vi "TWM Measure.vi"(4 "TWM Status ref":refnum<vi>, 6 "TWM pipe":string, 8 "error in (no error)":errorcluster, 10 "TWM Measurement properties":T1={"Sampling frequency (Hz)"=500000.0, "Record length (multiples of period)"=1000.0, "Signal amplitude (V)"=4.5, "Measurement frequency (Hz)"=1000.0, "Calculate RMS from samples"=FALSE, "Algorithm"="TWM-WFFT", "Quantity"="rms", "Measurement path"=""} {"Measurement frequency (Hz)" format="%#_3p"; "Record length (multiples of period)" format="%#_3p"; "Sampling frequency (Hz)" format="%#_3p"}, 11 "TWM handle":i32) -> (0 "error out":errorcluster, 1 "TWM result as number":dbl[][](array[numeric]), 2 "TWM result as string":string[][](array[string]), 3 "TWM handle out":i32)   [LabVIEW 2020]
doc: "Set TWM measurement, initiate TWM measurement, wait for results if needed, reset connection if error."
uses:
  Type definitions/Sampling properties.ctl
  external libraries/TWM-1.8.7.0-client/TWM Client Quantity Record.ctl
  external libraries/TWM-1.8.7.0-client/TWM Client.lvlib
  external libraries/varilib/varilib.lvlib
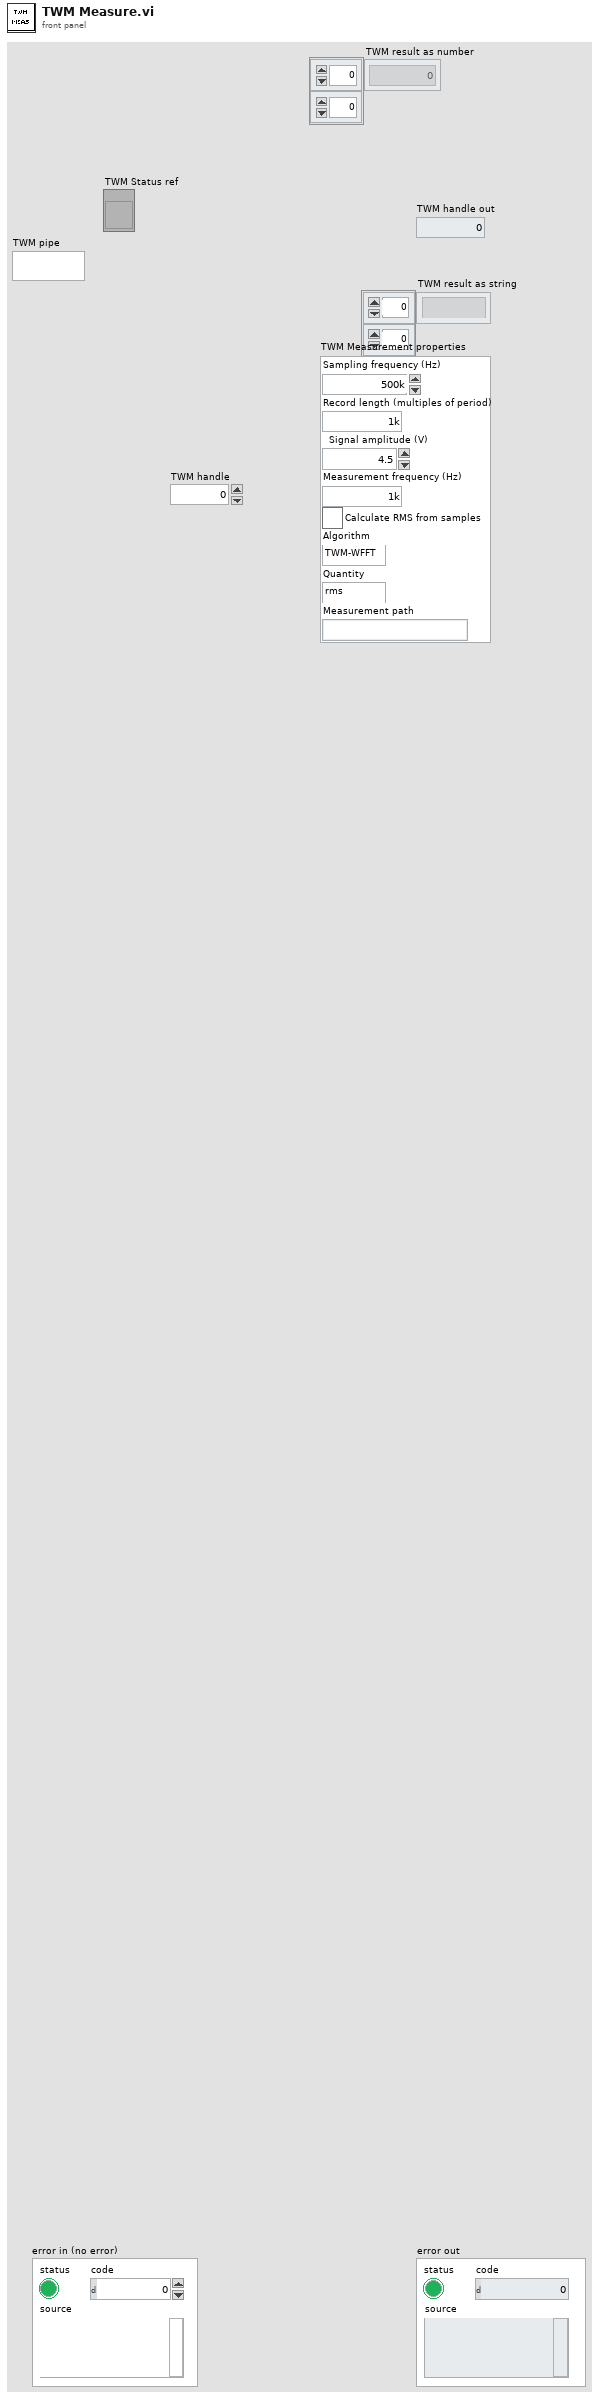
[diagram p1: front panel]
types:
  T1 = typedef "Sampling properties.ctl" = cluster{"Sampling frequency (Hz)":dbl, "Record length (multiples of period)":dbl, "Signal amplitude (V)":dbl, "Measurement frequency (Hz)":dbl, "Calculate RMS from samples":bool, "Algorithm":string, "Quantity":string, "Measurement path":string}
  T2 = typedef "TWM Client.lvlib/TWM Client Quantity Record.ctl" = cluster{"val":dbl[], "unc":dbl[], "name":string, "is valid?":bool, "has unc?":bool, "numel":i32, "ua":dbl[], "is phase?":bool, "is amplitude?":bool, "description":string, "phase tag":string, "num format":string, "is string?":bool, "string value":string}
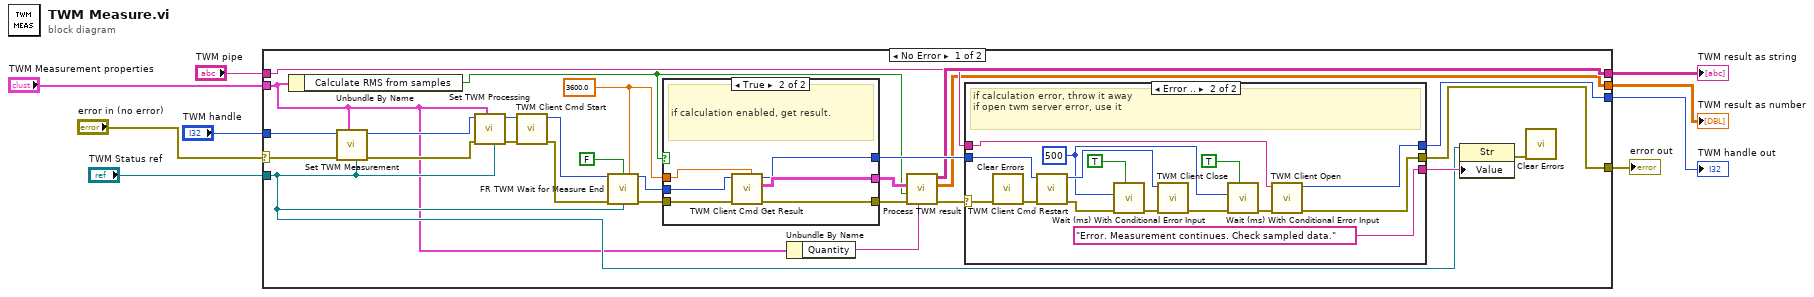
[diagram p0: block diagram]
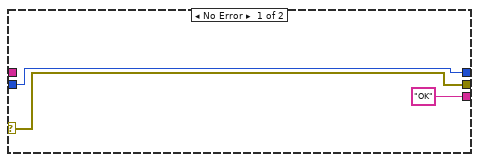
[diagram p2: hidden frame]
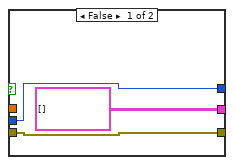
[diagram p3: hidden frame]
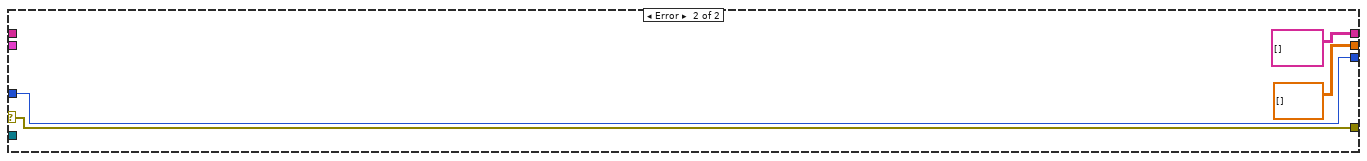
[diagram p4: hidden frame]
diagram:
  n1 = case shown="No Error" "error in (no error)" {
    selector: "error in (no error)" -> [w12 w67]
    tunnel: [w32 w66] -> w9
    tunnel: [w28 w67] -> w8
    tunnel: [w25 string[][] [] ("TWM result as string")] -> w7
    tunnel: "TWM handle" -> [w20 w66]
    tunnel: "TWM Measurement properties" -> [w11 _]
    tunnel: "TWM Status ref" -> [w16 _]
    tunnel: "TWM pipe" -> [w15 _]
    tunnel: [w14 dbl[][] [] ("TWM result as number")] -> w2
    frame No Error {
      w33 = 3600.0 ("timeout [s] (10s)")
      n2 = Unbundle By Name(w11) -> ("Calculate RMS from samples"=w17:bool)
      n3 = call "Set TWM Measurement.vi"("status ref (none)"=w16, "TWM Measurement properties"=w11, "error in"=w12, "TWM handle"=w20) -> ("error out"=w21:errorcluster, "TWM handle out"=w24:i32)  [unwired: 6 in]
      n4 = call "Set TWM Processing.vi"("status ref (none)"=w16, "TWM Measurement properties"=w11, "error in"=w21, "handle"=w24) -> ("error out"=w22:errorcluster, "handle out"=w23:i32)  [unwired: 6 in]
      n5 = call "TWM Client Cmd Start.vi"("error in"=w22, "handle"=w23) -> ("error out"=w18:errorcluster, "handle out"=w19:i32)  [unwired: 8 in]
      n6 = call "FR TWM Wait for Measure End.vi"("handle"=w19, "Obtain results? (False)"=FALSE, "timeout [s] (10s)"=w33, "error in"=w18, "status ref (none)"=w16) -> ("handle out"=w30:i32, "error out"=w29:errorcluster)  [unwired: 6 in, 3 out]
      n7 = case shown="True" w17 {
        tunnel: [T2[][] [] ("result data") w63] -> w26
        tunnel: w30 -> [w56 w62]
        tunnel: w29 -> [w55 w61]
        tunnel: [w56 w60] -> w31
        tunnel: w33 -> [_ w59]
        tunnel: [w55 w58] -> w34
        frame False {
        }
        frame True {
          # "if calculation enabled, get result."
          n8 = call "TWM Client Cmd Get Result.vi"("timeout [s] (10s)"=w59, "error in"=w61, "handle"=w62) -> ("error out"=w58:errorcluster, "result data"=w63:T2[][], "handle out"=w60:i32)  [unwired: 5 in, 1 out]
        }
      }
      n9 = Unbundle By Name(w11) -> ("Quantity"=w10:string)
      n10 = call "Process TWM result.vi"("Quantity to read"=w10, "error from TWM get result"=w34, "Calculate RMS from samples"=w17, "TWM result"=w26) -> ("error out"=w35:errorcluster, "TWM result as number"=w14:dbl[][], "TWM result as string"=w25:string[][])  [unwired: 5 in]
      n11 = case shown="Error .." w35 {
        selector: w35 -> [w39 w54]
        tunnel: [w39 w50] -> w28
        tunnel: w31 -> [w38 w53]
        tunnel: [w38 w49] -> w32
        tunnel: ["OK" ("Value") "Error. Measurement continues. Check sampled data." ("Value")] -> w36
        tunnel: w15 -> [_ w40]
        frame No Error {
        }
        frame Error {
          w42 = u32 500 ("milliseconds to wait")
          # "if calculation error, throw it away\nif open twm server error, use it"
          n12 = call <vilib>:"Clear Errors.vi"("error in (no error)"=w54) -> ("error out"=w52:errorcluster)  [unwired: 5 in, 1 out]
          n13 = call "TWM Client Cmd Restart.vi"("error in"=w52, "handle"=w53) -> ("error out"=w48:errorcluster, "handle out"=w51:i32)  [unwired: 8 in]
          n14 = call "Wait (ms) With Conditional Error Input.vi"("wait if error (F)"=TRUE, "error in (no error)"=w48, "milliseconds to wait"=w42) -> ("error out"=w47:errorcluster)  [unwired: 7 in, 1 out]
          n15 = call "TWM Client Close.vi"("error in"=w47, "handle in"=w51) -> ("error out"=w46:errorcluster)  [unwired: 9 in]
          n16 = call "Wait (ms) With Conditional Error Input.vi"("wait if error (F)"=TRUE, "error in (no error)"=w46, "milliseconds to wait"=w42) -> ("error out"=w45:errorcluster)  [unwired: 7 in, 1 out]
          n17 = call "TWM Client Open.vi"("error in"=w45, "pipe name"=w40) -> ("error out"=w50:errorcluster, "handle out"=w49:i32)  [unwired: 8 in]
        }
      }
      n18 = property class="Str"(reference=w16, "Value"=w36) -> (error out=w13:errorcluster)  [unwired: 1 in, 1 out]
      n19 = call <vilib>:"Clear Errors.vi"("error in (no error)"=w13) -> ()  [unwired: 5 in, 2 out]
    }
    frame Error {
    }
  }
  "TWM handle out" <- w9
  "error out" <- w8
  "TWM result as string" <- w7
  "TWM result as number" <- w2
